vi "ASS Timer (SubVI).vi"(0 "STOP Case":T1(ring), 4 "STOP":refnum<vi>, 5 "Next Case":T1(ring), 6 "Time":refnum<vi>, 7 "Light":refnum<vi>, 8 "Numeric":dbl, 9 "Vehicle Out Of Position":refnum<vi>, 10 "Current Case":T1(ring), 11 "Switch":refnum<vi>) -> (3 "Case Out":T1(ring))   [LabVIEW 2019]
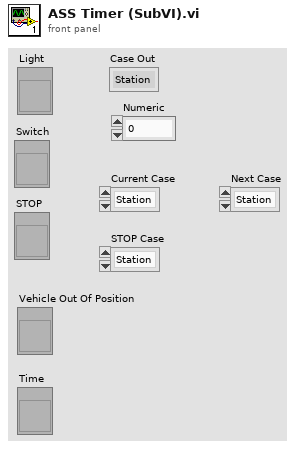
[diagram p1: front panel]
types:
  T1 = enum16{"Station", "Under Body", "Main Body", "Air Dry", "Report", "Stop"}
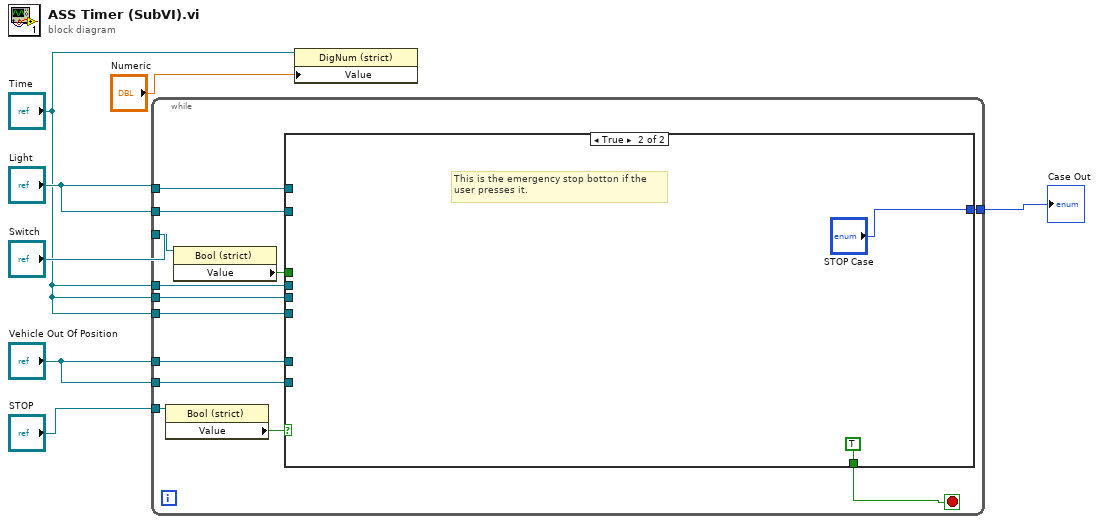
[diagram p0: block diagram]
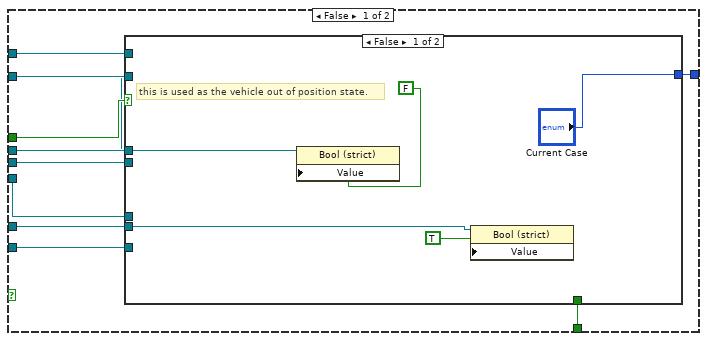
[diagram p2: hidden frame]
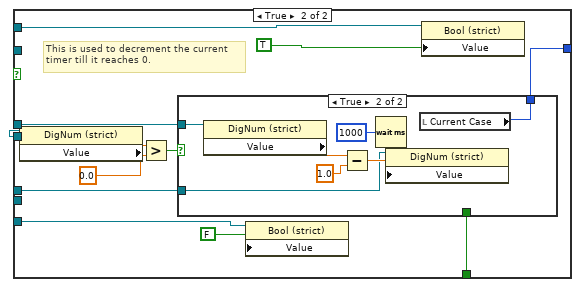
[diagram p3: hidden frame]
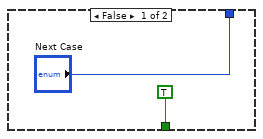
[diagram p4: hidden frame]
diagram:
  n1 = while {
    tunnel: [w19] -> w7
    tunnel: "Light" -> [w18]
    tunnel: "Vehicle Out Of Position" -> [w17]
    tunnel: "Light" -> [w16]
    tunnel: "Time" -> [w15]
    tunnel: "Time" -> [w14]
    tunnel: "Time" -> [w13]
    tunnel: "Vehicle Out Of Position" -> [w12]
    tunnel: "Switch" -> [w9]
    tunnel: "STOP" -> [w10]
    stop <- w20 stop-if-true
    n2 = property class="Bool (strict)"(reference=w10) -> ("Value"=w11:bool)  [unwired: 1 in, 2 out]
    n3 = property class="Bool (strict)"(reference=w9) -> ("Value"=w8:bool)  [unwired: 1 in, 2 out]
    n4 = case shown="True" w11 {
      tunnel: [w30 TRUE] -> w20
      tunnel: [w29 "STOP Case"] -> w19
      tunnel: w18 -> [w28 _]
      tunnel: w17 -> [w27 _]
      tunnel: w16 -> [w26 _]
      tunnel: w15 -> [w25 _]
      tunnel: w14 -> [w24 _]
      tunnel: w13 -> [w23 _]
      tunnel: w12 -> [w22 _]
      tunnel: w8 -> [w21 _]
      frame False {
        n5 = case shown="False" w21 {
          tunnel: [_ w46] -> w30
          tunnel: ["Current Case" w41] -> w29
          tunnel: w28 -> [w33 _]
          tunnel: w27 -> [w32 _]
          tunnel: w26 -> [_ w40]
          tunnel: w25 -> [_ w39]
          tunnel: w24 -> [_ w38]
          tunnel: w23 -> [_ w37]
          tunnel: w22 -> [_ w36]
          frame False {
            # "this is used as the vehicle out of position state."
            n6 = property class="Bool (strict)"(reference=w33, "Value"=FALSE ("Under Body Wash")) -> ()  [unwired: 1 in, 2 out]
            n7 = property class="Bool (strict)"(reference=w32, "Value"=TRUE ("Vehicle Out Of Position")) -> ()  [unwired: 1 in, 2 out]
          }
          frame True {
            # "This is used to decrement the current \ntimer till it reaches 0."
            n8 = property class="DigNum (strict)"(reference=w37) -> ("Value"=w45:dbl)  [unwired: 1 in, 2 out]
            n9 = Greater?(x=w45, y=0.0) -> (0:w43:bool)
            n10 = case shown="True" w43 {
              tunnel: [TRUE _] -> w46
              tunnel: ["Next Case" w50] -> w41
              tunnel: w39 -> [_ w52]
              tunnel: w38 -> [_ w51]
              frame False {
              }
              frame True {
                n11 = property class="DigNum (strict)"(reference=w51) -> ("Value"=w56:dbl)  [unwired: 1 in, 2 out]
                n12 = Subtract(x=w56, y=1.0) -> (x-y=w55:dbl)
                n13 = Wait (ms)(milliseconds to wait=u32 1000) -> ()  [unwired: 1 out]
                n14 = property class="DigNum (strict)"(reference=w52, "Value"=w55) -> ()  [unwired: 1 in, 2 out]
                n15 = local read "Current Case"() -> (w50:T1)
              }
            }
            n16 = property class="Bool (strict)"(reference=w36, "Value"=FALSE ("Vehicle Out Of Position")) -> ()  [unwired: 1 in, 2 out]
            n17 = property class="Bool (strict)"(reference=w40, "Value"=TRUE ("Under Body Wash")) -> ()  [unwired: 1 in, 2 out]
          }
        }
      }
      frame True {
        # "This is the emergency stop botton if the \nuser presses it."
      }
    }
  }
  "Case Out" <- w7
  n18 = property class="DigNum (strict)"(reference="Time", "Value"="Numeric") -> ()  [unwired: 1 in, 2 out]
